vi "GetIntFromDigitalCtrl.vi"(11 "int value ref":refnum<vi>) -> (3 "result":i32)   [LabVIEW 2018, in "Library-Ctrl.lvlib"]
uses:
  Library-Ctrl.lvlib
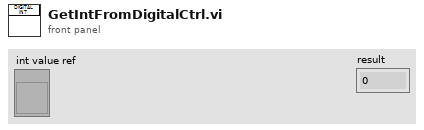
[diagram p1: front panel]
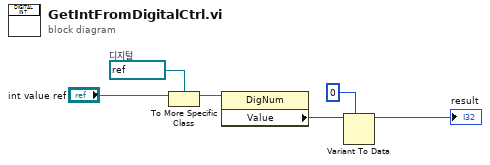
[diagram p0: block diagram]
diagram:
  w5 = refnum<vi> refnum  # 디지털
  n1 = To More Specific Class(target class=w5, reference="int value ref") -> (specific class reference=w4:refnum<vi>)  [unwired: 1 in, 1 out]
  n2 = property class="DigNum"(reference=w4) -> ("Value"=w3:variant)  [unwired: 1 in, 2 out]
  n3 = Variant To Data(type=0, Variant=w3) -> (data=→"result":i32)  [unwired: 1 in, 1 out]
